vi "TrigGatedProps.vi"(0 "task in":refnum<k24>, 5 "error in (no error)":errorcluster) -> (8 "When":i32, 9 "Hysteresis":i32, 10 "Position":i32, 11 "WindowBottom":dbl, 12 "Type":i32, 13 "WindowTop":dbl, 14 "task out":refnum<k24>, 15 "AnalogLevel":dbl, 16 "DigitalLevel":i32, 17 "HighThreshold":dbl, 18 "LowThreshold":dbl, 19 "error out":errorcluster)   [LabVIEW 2010]
uses:
  C:/Program Files/National Instruments/LabVIEW 2010/vi.lib/ULx/ULx_LV.dll
  Program Files/National Instruments/LabVIEW 2010/vi.lib/ULx/ULx_LV.dll
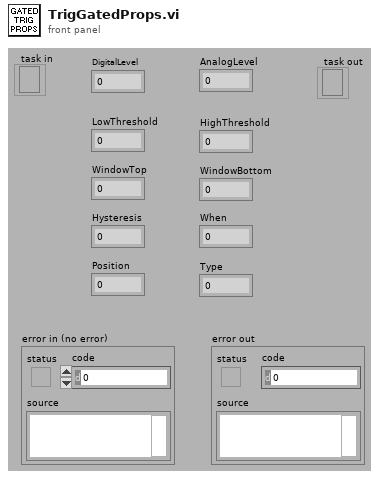
[diagram p1: front panel]
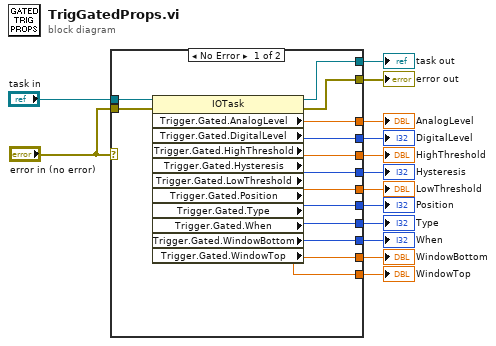
[diagram p0: block diagram]
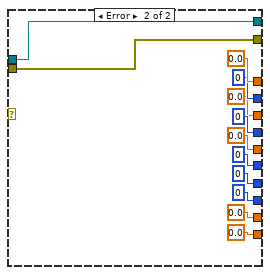
[diagram p2: hidden frame]
diagram:
  n1 = case shown="No Error" "error in (no error)" {
    tunnel: "task in" -> [w28 w40]
    tunnel: "error in (no error)" -> [w27 w35]
    tunnel: [w26 w40] -> w12
    tunnel: [w24 0.0 ("Trigger.Basic.AnalogLevel")] -> w1
    tunnel: [w23 0 ("Trigger.Basic.Type")] -> w2
    tunnel: [w22 0.0 ("Trigger.Gated.HighThreshold")] -> w3
    tunnel: [w21 0 ("Trigger.Basic.PretriggerCount")] -> w4
    tunnel: [w20 0.0 ("Trigger.Gated.LowThreshold")] -> w5
    tunnel: [w19 0 ("Trigger.Basic.Slope")] -> w6
    tunnel: [w18 0 ("Trigger.Gated.Type")] -> w7
    tunnel: [w17 0 ("Trigger.Gated.When")] -> w8
    tunnel: [w16 0.0 ("Trigger.Gated.WindowBottom")] -> w9
    tunnel: [w15 0.0 ("Trigger.Gated.WindowTop")] -> w10
    tunnel: [w25 w35] -> w11
    frame No Error {
      n2 = property class="IOTask"(reference=w28, error in=w27) -> (reference out=w26:refnum<k24>, error out=w25:errorcluster, "Trigger.Gated.AnalogLevel"=w24:dbl, "Trigger.Gated.DigitalLevel"=w23:i32, "Trigger.Gated.HighThreshold"=w22:dbl, "Trigger.Gated.Hysteresis"=w21:i32, "Trigger.Gated.LowThreshold"=w20:dbl, "Trigger.Gated.Position"=w19:i32, "Trigger.Gated.Type"=w18:i32, "Trigger.Gated.When"=w17:i32, "Trigger.Gated.WindowBottom"=w16:dbl, "Trigger.Gated.WindowTop"=w15:dbl)
    }
    frame Error {
    }
  }
  "task out" <- w12
  "error out" <- w11
  "WindowTop" <- w10
  "WindowBottom" <- w9
  "When" <- w8
  "Type" <- w7
  "Position" <- w6
  "LowThreshold" <- w5
  "Hysteresis" <- w4
  "HighThreshold" <- w3
  "DigitalLevel" <- w2
  "AnalogLevel" <- w1
